vi "Set_Parameter_Instrument (Json).vi"(8 "error in (no error)":errorcluster caption="entrée d'erreur (pas d'erreur)", 10 "Parameter (Json)":string, 11 "Nodon_Get_Power en entrée":refnum<class "Nodon_Get_Power.lvclass">) -> (0 "error out":errorcluster caption="sortie d'erreur", 3 "Nodon_Get_Power en sortie":refnum<class "Nodon_Get_Power.lvclass">)   [LabVIEW 2020, in "Library Test.lvlib" / "Nodon_Get_Power.lvclass"]
uses:
  Nodon_Get_Power.lvclass
  C:/Users/ngarcin/OneDrive - Altyor/Standard TB/Class/Test/Test (Default)/Test (Default).lvclass
  JSON API/JSON Value/Set from JSON string.vi
  Nodon_Send_Command_UART.lvclass
  JSON API/JSON Value/JSON Value.lvclass
  Nodon_Get_Power.lvclass/Nodon_Get_Power.ctl
  JSON API/Variant JSON/Variant JSON.lvlib
  JSON API/Get Polymorphic/JSON GetSet.lvlib
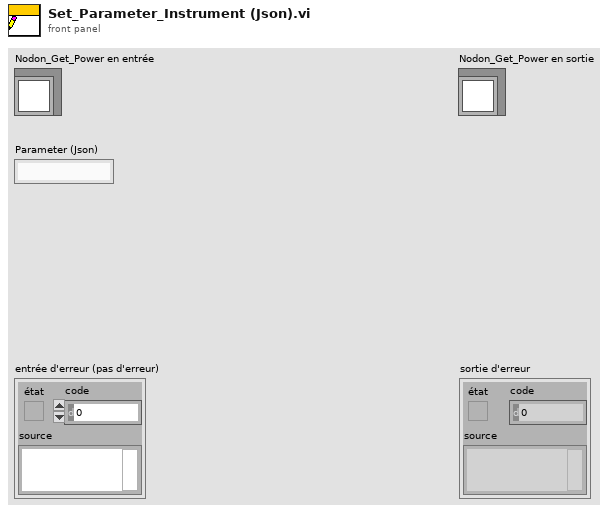
[diagram p1: front panel]
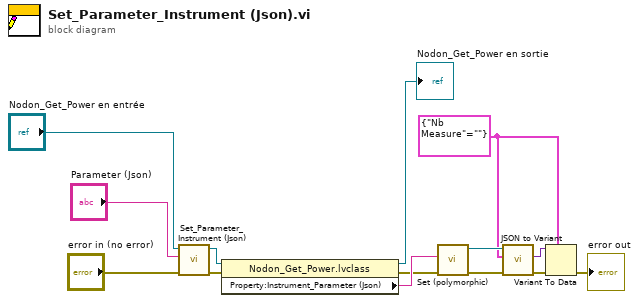
[diagram p0: block diagram]
diagram:
  w5 = cluster{"Nb Measure":string} {"Nb Measure"=""}
  n1 = call-parent "Set_Parameter_Instrument (Json).vi"("error in (no error)"="error in (no error)", "Parameter (Json)"="Parameter (Json)", "Test (Default) en entrée"="Nodon_Get_Power en entrée") -> ("error out"=w3:errorcluster, "Test (Default) en sortie"=w4:refnum<class "Nodon_Get_Power.lvclass">)  [unwired: 7 in]
  n2 = property class="Nodon_Get_Power.lvclass"(reference=w4, error in=w3) -> (reference out=→"Nodon_Get_Power en sortie":refnum<class "Nodon_Get_Power.lvclass">, error out=w6:errorcluster, "Property:Instrument_Parameter (Json)"=w7:string)
  n3 = call-poly "Set (polymorphic).vi"("error in (no error)"=w6, "JSON stream"=w7) -> ("error out"=w9:errorcluster, "JSON Value out"=w11:refnum<class "JSON Value.lvclass">)  [unwired: 7 in, 1 out]
  n4 = call "JSON to Variant.vi"("error in (no error)"=w9, "Variant (Data Type)"=w5, "JSON Value"=w11) -> ("error out"=w10:errorcluster, "Variant out"=w8:variant)  [unwired: 7 in]
  n5 = Variant To Data(error in=w10, type=w5, Variant=w8) -> (error out=→"error out":errorcluster)  [unwired: 1 out]
